vi "Begin.vi"(8 "error in":errorcluster) -> (0 "error out":errorcluster)   [LabVIEW 2017]
doc: "Called before other user functions, this VI is expected to open initial I/O refnums, load in file data, and do all program initialization. Notice that the <B>error out</B> terminal is simply used for data flow. Wiring it to other structures or subVIs ensures that this VI runs first."
uses:
  <vilib>/Rock Robotics/WPI/DriverStation/WPI_DriverStationRobotMode2.ctl
  <vilib>/Rock Robotics/WPI/Joystick/WPI_JoystickDeviceEnum.ctl
  <vilib>/Rock Robotics/SystemInterfaces/DIO/FPGA_DIOPWMChannel.ctl
  <vilib>/Rock Robotics/WPI/SafetyOutput/WPI_SafetyOutputConfigMenu.ctl
  <vilib>/Rock Robotics/WPI/Solenoid/WPI_SolenoidChannel.ctl
  <vilib>/Rock Robotics/SystemInterfaces/DIO/FPGA_DIORelayChannel.ctl
  <vilib>/Rock Robotics/WPI/Relay/WPI_RelayDirection.ctl
  Robot Global Data.vi
  <vilib>/Rock Robotics/Network Tables/NT Write String Array.vi
  <vilib>/Rock Robotics/WPI/RobotDrive/WPI_RobotDriveOpen4MotorWithVictorSP.vi
  <vilib>/Rock Robotics/WPI/Solenoid/WPI_SolenoidOpenDouble.vi
  <vilib>/Rock Robotics/WPI/MotorControl/WPI_MotorControlOpen VictorSP.vi
  <vilib>/Rock Robotics/WPI/MotorControl/WPI_MotorControlOpen SPARK.vi
  <vilib>/Rock Robotics/WPI/MotorControl/WPI_MotorControlOpen TalonSRX.vi
  <vilib>/Rock Robotics/WPI/Utilities/WPI_GetSetVariantRefNum.vi
  <vilib>/Rock Robotics/WPI/Counter/WPI_CounterDigitalInputToDigitalSource.vi
  <vilib>/Rock Robotics/SystemInterfaces/DIO/FPGA_DIOChannel.ctl
  <vilib>/Rock Robotics/WPI/ThirdParty/Sensors/ADIS16448 IMU/ADIS16448_IMU.lvlib
panel:
  in  "Invert Motor Encoders?":bool
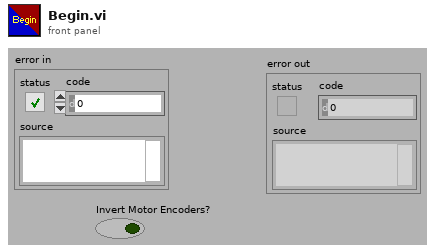
[diagram p1: front panel]
types:
  T1 = typedef "FPGA_DIOPWMChannel.ctl" = enum8{"PWM 0", "PWM 1", "PWM 2", "PWM 3", "PWM 4", "PWM 5", "PWM 6", "PWM 7", "PWM 8", "PWM 9", "PWM MXP 0", "PWM MXP 1", "PWM MXP 2", "PWM MXP 3", "PWM MXP 4", "PWM MXP 5", "PWM MXP 6", "PWM MXP 7", "PWM MXP 8", "PWM MXP 9", "Invalid"}
  T2 = typedef "WPI_RelayDirection.ctl" = enum16{"Both directions", "Forward only", "Reverse only"}
  T3 = typedef "FPGA_DIORelayChannel.ctl" = enum8{"Relay 0", "Relay 1", "Relay 2", "Relay 3", "Invalid"}
  T4 = typedef "WPI_SolenoidChannel.ctl" = enum8{"Solenoid 0", "Solenoid 1", "Solenoid 2", "Solenoid 3", "Solenoid 4", "Solenoid 5", "Solenoid 6", "Solenoid 7", "Invalid"}
  T5 = typedef "WPI_SafetyOutputConfigMenu.ctl" = enum16{"Enable", "Disable"}
  T6 = typedef "WPI_JoystickDeviceEnum.ctl" = enum16{"USB 0", "USB 1", "USB 2", "USB 3", "USB 4", "USB 5"}
  T7 = typedef "WPI_DriverStationRobotMode2.ctl" = enum16{"Autonomous Disabled", "Autonomous Enabled", "Teleop Disabled", "Teleop Enabled", "Disconnected", "Finish", "Test Disabled", "Test Enabled", "Emergency Stopped"}
  T8 = typedef "WPI_MotorControlDeviceRef.ctl" = cluster{"DeviceStatus":errorcluster, "Type":T9, "PWM":cluster{"PWM Channel":T1, "DeadBand":T10}, "CAN":cluster{"Device Number":u8, "SetOutput VI Ref":variant, "GetOutput VI Ref":variant, "Enable VI Ref":variant, "Disable VI Ref":variant, "Data":variant}, "Invert":bool, "DIO PWM":cluster{"PWM \"Enable\" Channel":T1, "DIOChannel":T11, "PWM Rate":dbl}}
  T9 = typedef "WPI_MotorControlType.ctl" = enum16{"PWM", "CAN", "DIO PWM"}
  T10 = typedef "WPI_PWMDeadband.ctl" = cluster{"Name":string, "maxPositivePwm":i32, "minPositivePwm":i32, "centerPwm":i32, "maxNegativePwm":i32, "minNegativePwm":i32, "angularRange":u16}
  T11 = typedef "FPGA_DIOChannel.ctl" = enum8{"DIO 0", "DIO 1", "DIO 2", "DIO 3", "DIO 4", "DIO 5", "DIO 6", "DIO 7", "DIO 8", "DIO 9", "DIO MXP 0", "DIO MXP 1", "DIO MXP 2", "DIO MXP 3", "DIO MXP 4", "DIO MXP 5", "DIO MXP 6", "DIO MXP 7", "DIO MXP 8", "DIO MXP 9", "DIO MXP 10", "DIO MXP 11", "DIO MXP 12", "DIO MXP 13", "DIO MXP 14", "DIO MXP 15", "SPI Port CS1", "SPI Port CS2", "SPI Port CS3", "SPI Port MISO", "SPI Port MOSI", "Invalid"}
  T12 = typedef "WPI_RobotDriveDevRef.ctl" = cluster{"DevStatus":errorcluster, "Motors[]":T8[], "Square Inputs":bool, "Max Output":dbl}
  T13 = typedef "WPI_CompressorDevRef.ctl" = cluster{"DevStatus":errorcluster, "Pneumatics Control Module":u8}
  T14 = typedef "WPI_RelayDevRef.ctl" = cluster{"DevStatus":errorcluster, "Relay Channel":T3, "Relay Direction":T2}
  T15 = typedef "ADIS16448_IMU.lvlib/ADI_IMU_ADIS16448_IMUDevRef.ctl" = cluster{"DevStatus":errorcluster, "Handle":i32, "SPI Bus":T16, "Device Found":bool, "Device Ready":bool, "Yaw Axis":enum16{"X", "Y", "Z"}, "AHRS Algorithm":enum16{"Complementary", "Madgwick"}, "Serial":u16, "Lot ID 2":u16, "Lot ID 1":u16, "Bytes Per Sample":u16, "Calibrate On Open?":bool}
  T16 = typedef "spi_bus.ctl" = enum16{"SPI On-Board, CS0", "SPI On-Board, CS1", "SPI On-Board, CS2", "SPI On-Board, CS3", "SPI MXP", "Invalid"}
  T17 = typedef "WPI_SolenoidDevRef.ctl" = cluster{"DevStatus":errorcluster, "Pneumatics Control Module":u8, "Forward Solenoid Channel":T4, "Reverse Solenoid Channel":T4}
  T18 = typedef "WPI_JoystickDevRef.ctl" = cluster{"Device":T6}
  T19 = typedef "WPI_DigitalInputDevRef.ctl" = cluster{"DevStatus":errorcluster, "DIO Channel":T11}
  T20 = typedef "FPGA_CounterEncoderSourceConvertionLVSourceType.ctl" = cluster{"DevStatus":errorcluster, "AnalogTriggerMode?":bool, "DigitalMode":cluster{"DIO Channel":T21}, "AnalogTriggerMode":cluster{"AnalogTriggerIndex":T22, "OutputType":T23}}
  T21 = typedef "FPGA_DIODigitalSourceChannel.ctl" = enum8{"DIO 0", "DIO 1", "DIO 2", "DIO 3", "DIO 4", "DIO 5", "DIO 6", "DIO 7", "DIO 8", "DIO 9", "DIO MXP 0", "DIO MXP 1", "DIO MXP 2", "DIO MXP 3", "DIO MXP 4", "DIO MXP 5", "DIO MXP 6", "DIO MXP 7", "DIO MXP 8", "DIO MXP 9", "DIO MXP 10", "DIO MXP 11", "DIO MXP 12", "DIO MXP 13", "DIO MXP 14", "DIO MXP 15", "Disabled"}
  T22 = typedef "FPGA_AnalogTriggerIndex.ctl" = enum8{"Trig 0", "Trig 1", "Trig 2", "Trig 3", "Trig 4", "Trig 5", "Trig 6", "Trig 7", "Invalid"}
  T23 = typedef "FPGA_AnalogTriggerOutType.ctl" = enum16{"InWindow", "TriggerState", "Rising", "Falling"}
  T24 = typedef "WPI_EncoderDevRef.ctl" = cluster{"DevStatus":errorcluster, "EncoderIndex":T25, "CounterIndex":T26, "DistancePerCount":dbl, "Decoding Type":T27}
  T25 = typedef "FPGA_EncoderIdx.ctl" = enum8{"Enc 0", "Enc 1", "Enc 2", "Enc 3", "Enc 4", "Enc 5", "Enc 6", "Enc 7", "Invalid"}
  T26 = typedef "FPGA_CounterCtrSystemIndex.ctl" = enum8{"Ctr 0", "Ctr 1", "Ctr 2", "Ctr 3", "Ctr 4", "Ctr 5", "Ctr 6", "Ctr 7", "Invalid"}
  T27 = typedef "WPI_EncoderType.ctl" = enum16{"1x", "2x", "4x"}
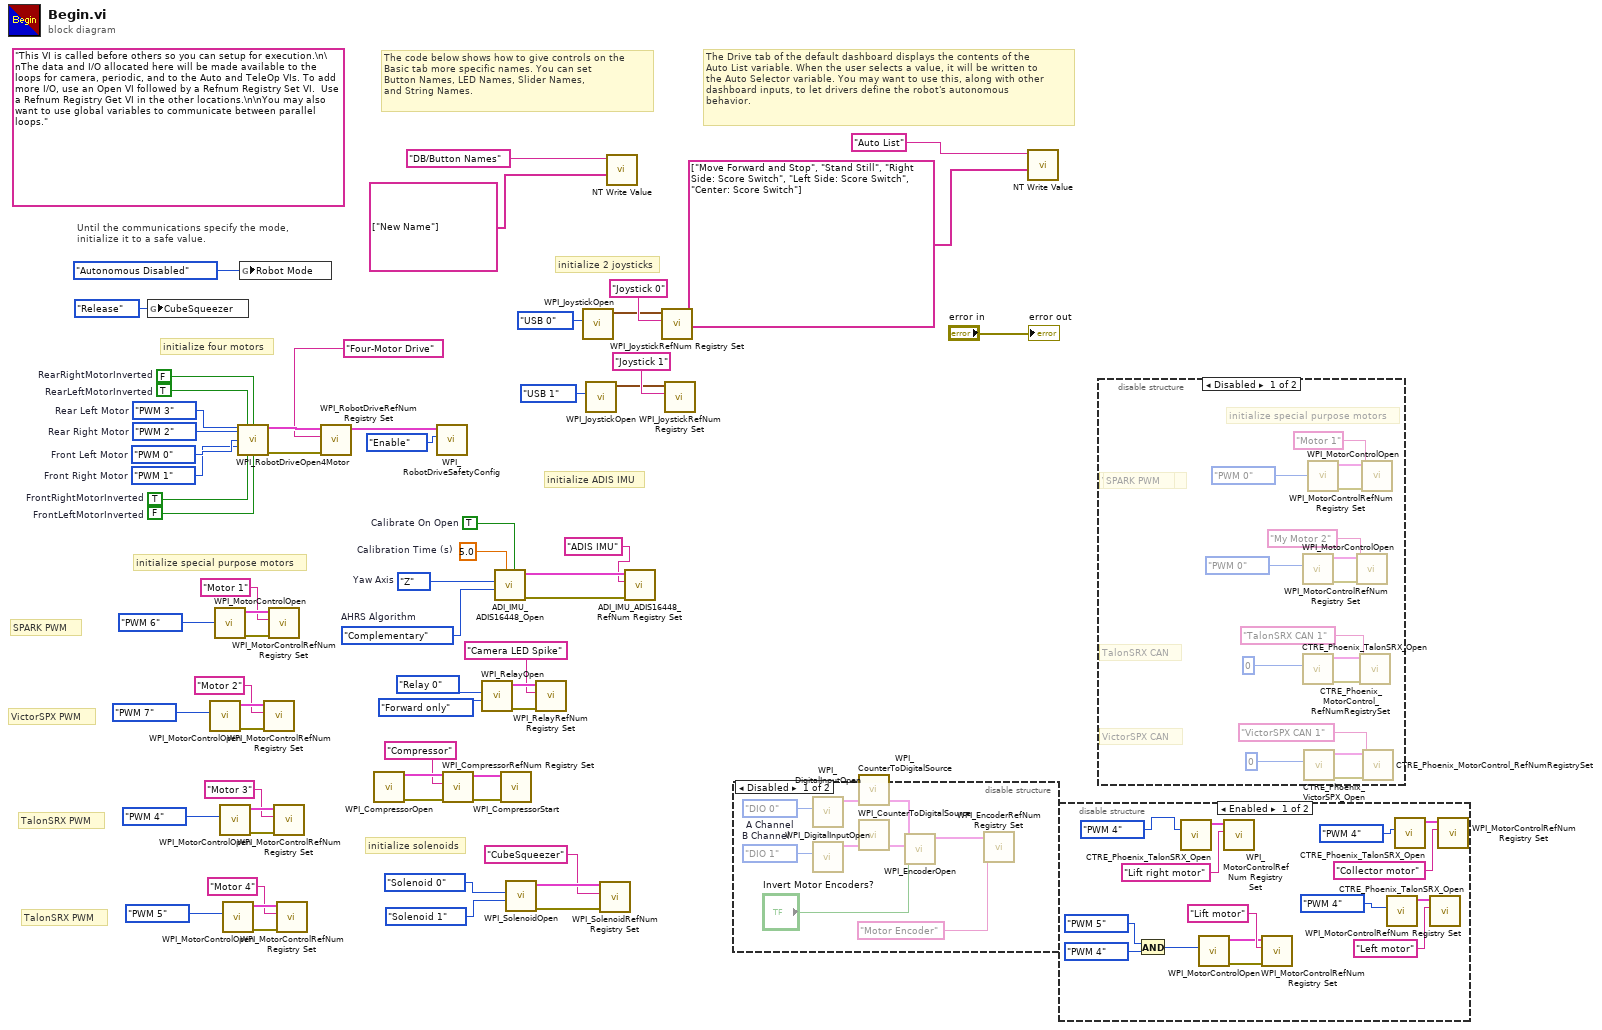
[diagram p0: block diagram]
diagram:
  w21 = TRUE  # Calibrate On Open
  w22 = 5.0  # Calibration Time (s)
  w23 = enum16{"Complementary", "Madgwick"}."Complementary"  # AHRS Algorithm
  w24 = enum16{"X", "Y", "Z"}."Z"  # Yaw Axis
  w41 = TRUE  # RearLeftMotorInverted
  w40 = FALSE  # RearRightMotorInverted
  w42 = FALSE  # FrontLeftMotorInverted
  w43 = TRUE  # FrontRightMotorInverted
  w44 = FPGA_DIOPWMChannel."PWM 1"  # Front Right Motor
  w45 = FPGA_DIOPWMChannel."PWM 0"  # Front Left Motor
  w46 = FPGA_DIOPWMChannel."PWM 2"  # Rear Right Motor
  w47 = FPGA_DIOPWMChannel."PWM 3"  # Rear Left Motor
  (unwired) "This VI is called before others so you can setup for execution.\n\nThe data and I/O allocated here will be made available to the loops for camera, periodic, and to the Auto and TeleOp VIs. To add more I/O, use an Open VI followed by a Refnum Registry Set VI.  Use a Refnum Registry Get VI in the other locations.\n\nYou may also want to use global variables to communicate between parallel loops."
  # "TalonSRX PWM"
  # "TalonSRX PWM"
  # "SPARK PWM"
  # "VictorSPX PWM"
  # "initialize special purpose motors"
  # "initialize ADIS IMU"
  # "initialize solenoids"
  # "initialize four motors"
  # "The Drive tab of the default dashboard displays the contents of the\nAuto List variable. When the user selects a value, it will be written to\nthe Auto Selector variable. You may want to use this, along with other\ndashboard inputs, to let drivers define the robot's autonomous\nbehavior."
  # "The code below shows how to give controls on the\nBasic tab more specific names. You can set\nButton Names, LED Names, Slider Names,\nand String Names."
  # "initialize 2 joysticks"
  # "Until the communications specify the mode,\ninitialize it to a safe value."
  n1 = global write "Robot Global Data.vi" "CubeSqueezer"(enum16{"Squeeze", "Release"}."Release" ("CubeSqueezer")) -> ()
  n2 = call-poly <vilib>:"WPI_MotorControlOpen.vi"("PWM Channel"=FPGA_DIOPWMChannel."PWM 7") -> ("error out"=w16:errorcluster, "MotorControlDeviceRef"=w15:T8)  [unwired: 9 in]
  n3 = call-poly <vilib>:"WPI_MotorControlOpen.vi"("PWM Channel"=FPGA_DIOPWMChannel."PWM 6") -> ("error out"=w14:errorcluster, "MotorControlDeviceRef"=w13:T8)  [unwired: 9 in]
  n4 = call-poly <vilib>:"WPI_MotorControlOpen.vi"("PWM Channel"=FPGA_DIOPWMChannel."PWM 4") -> ("error out"=w8:errorcluster, "MotorControlDeviceRef"=w7:T8)  [unwired: 9 in]
  n5 = call-poly <vilib>:"WPI_MotorControlOpen.vi"("PWM Channel"=FPGA_DIOPWMChannel."PWM 5") -> ("error out"=w4:errorcluster, "MotorControlDeviceRef"=w3:T8)  [unwired: 9 in]
  n6 = call-poly <vilib>:"WPI_RobotDriveOpen4Motor.vi"("Rear Left Motor"=w47, "Rear Left Motor Inverted"=w41, "Rear Right Motor Inverted"=w40, "Rear Right Motor"=w46, "Front Left Motor"=w45, "Front Right Motor"=w44, "Front Left Motor Inverted"=w43, "Front Right Motor Inverted"=w42) -> ("RobotDriveDevRef"=w52:T12, "error out"=w50:errorcluster)  [unwired: 6 in]
  n7 = global write "Robot Global Data.vi" "Robot Mode"(WPI_DriverStationRobotMode2."Autonomous Disabled" ("Robot Mode")) -> ()
  n8 = call <vilib>:"WPI_MotorControlRefNum Registry Set.vi"("error in (no error)"=w16, "refnum name"="Motor 2", "MotorControlDevRef"=w15) -> ()  [unwired: 7 in, 2 out]
  n9 = call <vilib>:"WPI_MotorControlRefNum Registry Set.vi"("error in (no error)"=w14, "refnum name"="Motor 1", "MotorControlDevRef"=w13) -> ()  [unwired: 7 in, 2 out]
  n10 = call <vilib>:"WPI_MotorControlRefNum Registry Set.vi"("error in (no error)"=w8, "refnum name"="Motor 3", "MotorControlDevRef"=w7) -> ()  [unwired: 7 in, 2 out]
  n11 = call <vilib>:"WPI_MotorControlRefNum Registry Set.vi"("error in (no error)"=w4, "refnum name"="Motor 4", "MotorControlDevRef"=w3) -> ()  [unwired: 7 in, 2 out]
  n12 = call <vilib>:"WPI_RobotDriveRefNum Registry Set.vi"("error in (no error)"=w50, "refnum name"="Four-Motor Drive", "RobotDriveDevRef"=w52) -> ("RobotDriveDevRef"=w49:T12)  [unwired: 1 in, 7 out]
  n13 = call <vilib>:"WPI_CompressorOpen.vi"() -> ("CompressorDevRef"=w31:T13, "error out"=w32:errorcluster)  [unwired: 14 in]
  n14 = call <vilib>:"WPI_RobotDriveSafetyConfig.vi"("mode"=WPI_SafetyOutputConfigMenu."Enable", "RobotDriveDevRef"=w49) -> ()  [unwired: 8 in, 2 out]
  n15 = call <vilib>:"WPI_CompressorRefNum Registry Set.vi"("error in (no error)"=w32, "refnum name"="Compressor", "CompressorDevRef"=w31) -> ("error out"=w30:errorcluster, "CompressorDevRef"=w29:T13)  [unwired: 7 in]
  n16 = call <vilib>:"WPI_RelayOpen.vi"("Relay Direction"=WPI_RelayDirection."Forward only", "Relay Channel"=FPGA_DIORelayChannel."Relay 0") -> ("error out"=w34:errorcluster, "RelayDevRef"=w33:T14)  [unwired: 8 in]
  n17 = call <vilib>:"ADI_IMU_ADIS16448_Open.vi"("Calibrate On Open"=w21, "Calibration Time (s)"=w22, "AHRS Algorithm"=w23, "Yaw Axis"=w24) -> ("error out"=w20:errorcluster, "ADI IMU DevRef Out"=w19:T15)  [unwired: 5 in, 1 out]
  n18 = call <vilib>:"WPI_CompressorStart.vi"("error in (no error)"=w30, "CompressorDevRef"=w29) -> ()  [unwired: 8 in, 2 out]
  n19 = call-poly <vilib>:"WPI_SolenoidOpen.vi"("Reverse Solenoid Channel"=WPI_SolenoidChannel."Solenoid 1" ("Extend Solenoid Channel"), "Forward Solenoid Channel"=WPI_SolenoidChannel."Solenoid 0" ("Retract Solenoid Channel")) -> ("error out"=w37:errorcluster, "SolenoidDevRef"=w36:T17)  [unwired: 2 in, 6 out]
  n20 = call <vilib>:"WPI_RelayRefNum Registry Set.vi"("error in (no error)"=w34, "refnum name"="Camera LED Spike", "RelayDevRef"=w33) -> ()  [unwired: 7 in, 2 out]
  n21 = call <vilib>:"WPI_JoystickOpen.vi"("JoystickDevice"=WPI_JoystickDeviceEnum."USB 0") -> ("JoystickDevRef"=w57:T18)  [unwired: 10 in]
  n22 = call <vilib>:"WPI_JoystickOpen.vi"("JoystickDevice"=WPI_JoystickDeviceEnum."USB 1") -> ("JoystickDevRef"=w54:T18)  [unwired: 10 in]
  n23 = call <vilib>:"WPI_SolenoidRefNum Registry Set.vi"("error in (no error)"=w37, "refnum name"="CubeSqueezer", "SolenoidDevRef"=w36) -> ()  [unwired: 7 in, 2 out]
  n24 = call-poly <vilib>:"NT Write Value.vi"("String Array"=string[] ["New Name"], "Name"="DB/Button Names") -> ()  [unwired: 9 in, 1 out]
  n25 = call <vilib>:"ADI_IMU_ADIS16448_RefNum Registry Set.vi"("error in (no error)"=w20, "refnum name"="ADIS IMU", "ADI IMU DevRef"=w19) -> ()  [unwired: 7 in, 2 out]
  n26 = call <vilib>:"WPI_JoystickRefNum Registry Set.vi"("refnum name"="Joystick 0", "JoystickDevRef"=w57) -> ()  [unwired: 8 in, 2 out]
  n27 = call <vilib>:"WPI_JoystickRefNum Registry Set.vi"("refnum name"="Joystick 1", "JoystickDevRef"=w54) -> ()  [unwired: 8 in, 2 out]
  n28 = disable-structure shown="Disabled" {
    frame Disabled {
      w73 = FPGA_DIOChannel."DIO 1"  # B Channel
      w72 = FPGA_DIOChannel."DIO 0"  # A Channel
      n29 = call <vilib>:"WPI_DigitalInputOpen.vi"("DIO Channel"=w72) -> ("DigitalInputDevRef"=w69:T19)  [unwired: 1 in, 9 out]
      n30 = call <vilib>:"WPI_DigitalInputOpen.vi"("DIO Channel"=w73) -> ("DigitalInputDevRef"=w70:T19)  [unwired: 1 in, 9 out]
      n31 = call-poly <vilib>:"WPI_CounterToDigitalSource.vi"("DigitalInputDevRef"=w69) -> ("Digital Source"=w68:T20)  [unwired: 6 out]
      n32 = call-poly <vilib>:"WPI_CounterToDigitalSource.vi"("DigitalInputDevRef"=w70) -> ("Digital Source"=w71:T20)  [unwired: 6 out]
      n33 = call <vilib>:"WPI_EncoderOpen.vi"("Invert Direction (False)"="Invert Motor Encoders?", "BSource"=w71, "ASource"=w68) -> ("EncoderDevRef"=w67:T24)  [unwired: 5 in, 3 out]
      n34 = call <vilib>:"WPI_EncoderRefNum Registry Set.vi"("refnum name"="Motor Encoder", "EncoderDevRef"=w67) -> ()  [unwired: 8 in, 2 out]
    }
    frame Enabled {
    }
  }
  n35 = call-poly <vilib>:"NT Write Value.vi"("String Array"=string[] ["Move Forward and Stop", "Stand Still", "Right Side: Score Switch", "Left Side: Score Switch", "Center: Score Switch"], "Name"="Auto List") -> ()  [unwired: 9 in, 1 out]
  n36 = disable-structure shown="Enabled" {
    frame Enabled {
      n37 = And(x=FPGA_DIOPWMChannel."PWM 5" ("PWM Channel"), y=FPGA_DIOPWMChannel."PWM 4" ("PWM Channel")) -> (x .and. y?=w75:i32)
      n38 = call <vilib>:"CTRE_Phoenix_TalonSRX_Open.vi"("Device Number"=FPGA_DIOPWMChannel."PWM 4" ("PWM Channel")) -> ("CAN Talon SRX Ref"=w83:T8)  [unwired: 9 in, 1 out]
      n39 = call-poly <vilib>:"WPI_MotorControlOpen.vi"("PWM Channel"=w75) -> ("error out"=w74:errorcluster, "MotorControlDeviceRef"=w84:T8)  [unwired: 9 in]
      n40 = call <vilib>:"WPI_MotorControlRefNum Registry Set.vi"("refnum name"="Lift right motor", "MotorControlDevRef"=w83) -> ()  [unwired: 8 in, 2 out]
      n41 = call <vilib>:"WPI_MotorControlRefNum Registry Set.vi"("error in (no error)"=w74, "refnum name"="Lift motor", "MotorControlDevRef"=w84) -> ()  [unwired: 7 in, 2 out]
      n42 = call <vilib>:"CTRE_Phoenix_TalonSRX_Open.vi"("Device Number"=FPGA_DIOPWMChannel."PWM 4" ("PWM Channel")) -> ("CAN Talon SRX Ref"=w81:T8)  [unwired: 9 in, 1 out]
      n43 = call <vilib>:"CTRE_Phoenix_TalonSRX_Open.vi"("Device Number"=FPGA_DIOPWMChannel."PWM 4" ("PWM Channel")) -> ("CAN Talon SRX Ref"=w85:T8)  [unwired: 9 in, 1 out]
      n44 = call <vilib>:"WPI_MotorControlRefNum Registry Set.vi"("refnum name"="Left motor", "MotorControlDevRef"=w81) -> ()  [unwired: 8 in, 2 out]
      n45 = call <vilib>:"WPI_MotorControlRefNum Registry Set.vi"("refnum name"="Collector motor", "MotorControlDevRef"=w85) -> ()  [unwired: 8 in, 2 out]
    }
    frame Disabled {
    }
  }
  n46 = disable-structure shown="Disabled" {
    frame Disabled {
      # "SPARK PWM"
      # "VictorSPX PWM"
      # "VictorSPX CAN"
      # "TalonSRX CAN"
      # "initialize special purpose motors"
      n47 = call-poly <vilib>:"WPI_MotorControlOpen.vi"("PWM Channel"=FPGA_DIOPWMChannel."PWM 0") -> ("error out"=w100:errorcluster, "MotorControlDeviceRef"=w99:T8)  [unwired: 9 in]
      n48 = call <vilib>:"CTRE_Phoenix_TalonSRX_Open.vi"("Device Number"=u8 0) -> ("error out"=w102:errorcluster, "CAN Talon SRX Ref"=w101:T8)  [unwired: 9 in]
      n49 = call <vilib>:"CTRE_Phoenix_VictorSPX_Open.vi"("Device Number"=u8 0) -> ("error out"=w104:errorcluster, "CAN Talon SRX Ref"=w103:T8)  [unwired: 9 in]
      n50 = call-poly <vilib>:"WPI_MotorControlOpen.vi"("PWM Channel"=FPGA_DIOPWMChannel."PWM 0") -> ("error out"=w98:errorcluster, "MotorControlDeviceRef"=w97:T8)  [unwired: 9 in]
      n51 = call <vilib>:"WPI_MotorControlRefNum Registry Set.vi"("error in (no error)"=w100, "refnum name"="My Motor 2", "MotorControlDevRef"=w99) -> ()  [unwired: 7 in, 2 out]
      n52 = call <vilib>:"CTRE_Phoenix_MotorControl_RefNumRegistrySet.vi"("error in (no error)"=w102, "refnum name"="TalonSRX CAN 1", "PhoenixMotorControlDevRef"=w101) -> ()  [unwired: 7 in, 2 out]
      n53 = call <vilib>:"WPI_MotorControlRefNum Registry Set.vi"("error in (no error)"=w98, "refnum name"="Motor 1", "MotorControlDevRef"=w97) -> ()  [unwired: 7 in, 2 out]
      n54 = call <vilib>:"CTRE_Phoenix_MotorControl_RefNumRegistrySet.vi"("error in (no error)"=w104, "refnum name"="VictorSPX CAN 1", "PhoenixMotorControlDevRef"=w103) -> ()  [unwired: 7 in, 2 out]
    }
    frame Enabled {
    }
  }
  "error out" <- "error in"
